vi "cli main.vi"(11 "builder settings":T1) -> (0 "error out":errorcluster, 3 "GeneratedFiles":path[](array[path]))   [LabVIEW 2024]
uses:
  <vilib>/AppBuilder/AB_API/common/AB_API Version Number.ctl
  <vilib>/AppBuilder/AB_API/common/AB_API Version Information.ctl
  typedefs/builder settings.ctl
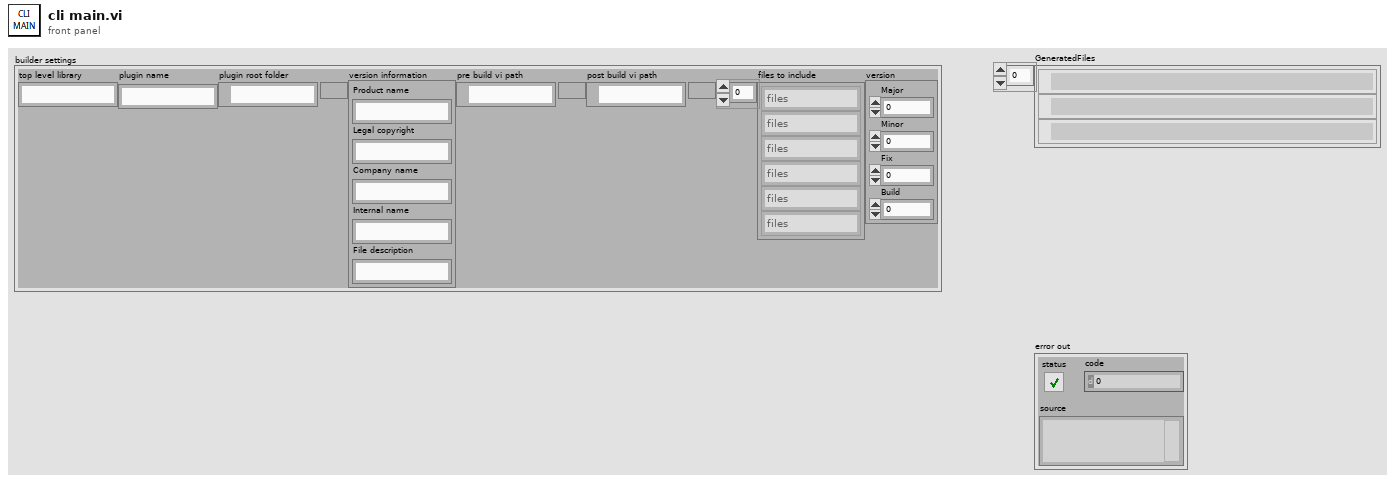
[diagram p1: front panel]
types:
  T1 = typedef "builder settings.ctl" = cluster{"top level library":string, "plugin name":string, "plugin root folder":path, "version information":T2, "pre build vi path":path, "post build vi path":path, "files to include":string[], "version":T3}
  T2 = typedef "AB_API Version Information.ctl" = cluster{"Product name":string, "Legal copyright":string, "Company name":string, "Internal name":string, "File description":string}
  T3 = typedef "AB_API Version Number.ctl" = cluster{"Major":u16, "Minor":u16, "Fix":u16, "Build":u16}
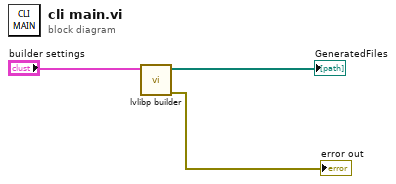
[diagram p0: block diagram]
diagram:
  n1 = call "lvlibp builder.vi"("builder settings"="builder settings") -> ("error out"=→"error out":errorcluster, "GeneratedFiles"=→"GeneratedFiles":path[])  [unwired: 7 in, 2 out]
